vi "quardrant distribution.vi"(9 "angle":dbl, 10 "input radial point":dbl) -> (0 "quardrant 4":dbl, 1 "quardrant 3":dbl, 2 "quardrant 2":dbl, 3 "quardrant 1":dbl)   [LabVIEW 2013]
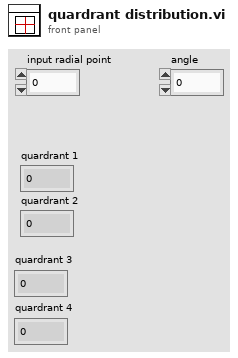
[diagram p1: front panel]
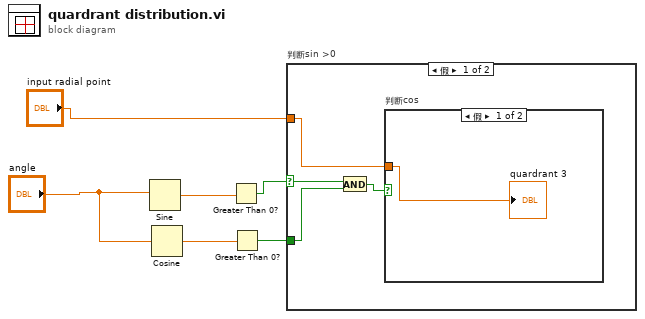
[diagram p0: block diagram]
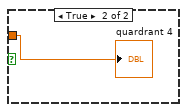
[diagram p2: hidden frame]
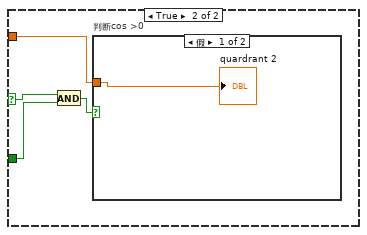
[diagram p3: hidden frame]
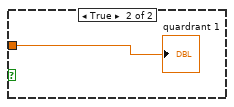
[diagram p4: hidden frame]
diagram:
  n1 = Sine(x="angle") -> (sin(x)=w6:dbl)
  n2 = Cosine(x="angle") -> (cos(x)=w5:dbl)
  n3 = Greater Than 0?(x=w6) -> (x > 0?=w4:bool)
  n4 = Greater Than 0?(x=w5) -> (x > 0?=w3:bool)
  n5 = case "判断sin >0" shown="假" w4 {
    selector: w4 -> [w10 w15]
    tunnel: w3 -> [w9 w16]
    tunnel: "input radial point" -> [w7 w13]
    frame False {
      n6 = And(x=w10, y=w9) -> (x .and. y?=w8:bool)
      n7 = case "判断cos" shown="假" w8 {
        tunnel: w7 -> [w11 w12]
        frame False {
          "quardrant 3" <- w11
        }
        frame True {
          "quardrant 4" <- w12
        }
      }
    }
    frame True {
      n8 = And(x=w15, y=w16) -> (x .and. y?=w14:bool)
      n9 = case "判断cos >0" shown="假" w14 {
        tunnel: w13 -> [w17 w18]
        frame False {
          "quardrant 2" <- w17
        }
        frame True {
          "quardrant 1" <- w18
        }
      }
    }
  }
